vi "LIDAR V2 Mem1 Manager.vi"(11 "Source Name":refnum<k21>="100 MHz Clock") -> ()   [LabVIEW 2013]
uses:
  <vilib>/Platform/TimedLoop/XDataNode/timing_clust.ctl
  <vilib>/Platform/TimedLoop/XDataNode/nitl_modes.ctl
  <vilib>/Platform/TimedLoop/XDataNode/wakeup.ctl
  <vilib>/rvi/DataTransferAndStorage/Container/Common/niFpgaContainerGetUniqueNameForEmu.vi
  <vilib>/rvi/DataTransferAndStorage/Container/Common/niFpgaContainerSetEmuInfo.vi
  <vilib>/rvi/eio/common/nirviEmuReportErrorAndStop.vi
  <vilib>/rvi/Emulation/niFpgaSctlEmulationGetInTimedLoop.vi
  <vilib>/rvi/Emulation/niFpgaEmulationReportErrorSimple.vi
  <vilib>/rvi/Emulation/niFpgaGetClockAttributes.vi
  <vilib>/rvi/Emulation/niFpgaCriticalErrorInLSC.vi
  <vilib>/rvi/DataTransferAndStorage/Container/Common/niFpgaContainerExecOnDevCompGetState.vi
  <vilib>/rvi/FIFO/Fifo_Resource/nirvififoEmulationReadFpgaImpl.vi
  <vilib>/rvi/interface/RandomDataEmulation/nirviRandomDataFPGAFIFO.vi
  <vilib>/rvi/interface/RandomDataEmulation/niFpgaRandomDataHandleErrors.vi
  <vilib>/rvi/Memory/Memory_Emulation/nirvimemoryFastEmulationFpgaImpl.vi
  <instcachedir>/0/nirvimemoryFastEmulationFpgaImpl_5FBAB50466BC4C939F684F8805638BFC.lvgen/nirvimemoryFastEmulationFpgaImpl_5FBAB50466BC4C939F684F8805638BFC_008.vi
  <vilib>/rvi/Memory/Memory_Emulation/nirvimemoryFastEmulation.vi
  <vilib>/rvi/Memory/Memory_Emulation/nirvimemoryEmulation.vi
  <vilib>/rvi/FIFO/Fifo_Resource/nirvififoEmulationWriteFpgaImpl.vi
  <vilib>/Platform/TimedLoop/XDataNode/XDataNode.xnode
  <vilib>/rvi/LocalResourceManager/LocalResourceManager.xnode
  <vilib>/rvi/DataTransferAndStorage/Container/XNode/niFpgaContainer.xnode
  <vilib>/rvi/FIFO/Fifo_Resource/niFpgaFifoEmulationRefIn.vi
  <vilib>/rvi/FIFO/Fifo_Resource/nirvififoEmulationRead.vi
  <vilib>/rvi/FXPMathLib/FxpAdd/XNode/nifxpmath_Add.xnode
  <vilib>/rvi/FIFO/Fifo_Resource/nirvififoEmulationWrite.vi
  <vilib>/Platform/TimedLoop/XDataNode/XDNodeRunTimeDep.lvlib
  <vilib>/rvi/FXPMathLib/sim/FxpSim.dll
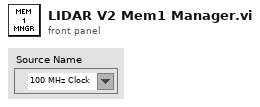
[diagram p1: front panel]
types:
  T1 = typedef "XDNodeRunTimeDep.lvlib/timing_clust.ctl" = cluster{"Expected End [f-1]":u64, "Actual End [f-1]":u64, "Finished Late? [f-1]":bool, "Expected End [i-1]":u64, "Actual End [i-1]":u64, "Finished Late? [i-1]":bool, "Expected Start [i]":u64, "Actual Start [i]":u64, "Expected Start [f]":u64, "Actual Start [f]":u64, "Source Name":string, "Structure Name":string, "Period":i64, "Deadline":i64, "Offset":i64, "Start":i64, "Priority":i32, "Timeout":i32, "Mode":T2, "Wakeup Reason":T3, "Error":errorcluster, "Source Type":string, "Secondary Source Type":string, "Global End Time":u64, "Global Start Time":u64, "Frame Duration":u64, "Iteration Duration":u64, "Assigned CPU":i32, "I/O Scan Engine Mode":u32}
  T2 = typedef "XDNodeRunTimeDep.lvlib/nitl_modes.ctl" = enum32{"No Change", "Process missed periods, maintain original phase", "Discard missed periods, maintain original phase", "Process missed periods, ignore original phase", "Discard missed periods, ignore original phase"}
  T3 = typedef "XDNodeRunTimeDep.lvlib/wakeup.ctl" = enum32{"Normal", "Aborted", "Asynchronous wakeup", "Timing source error", "Timed loop error", "Timeout"}
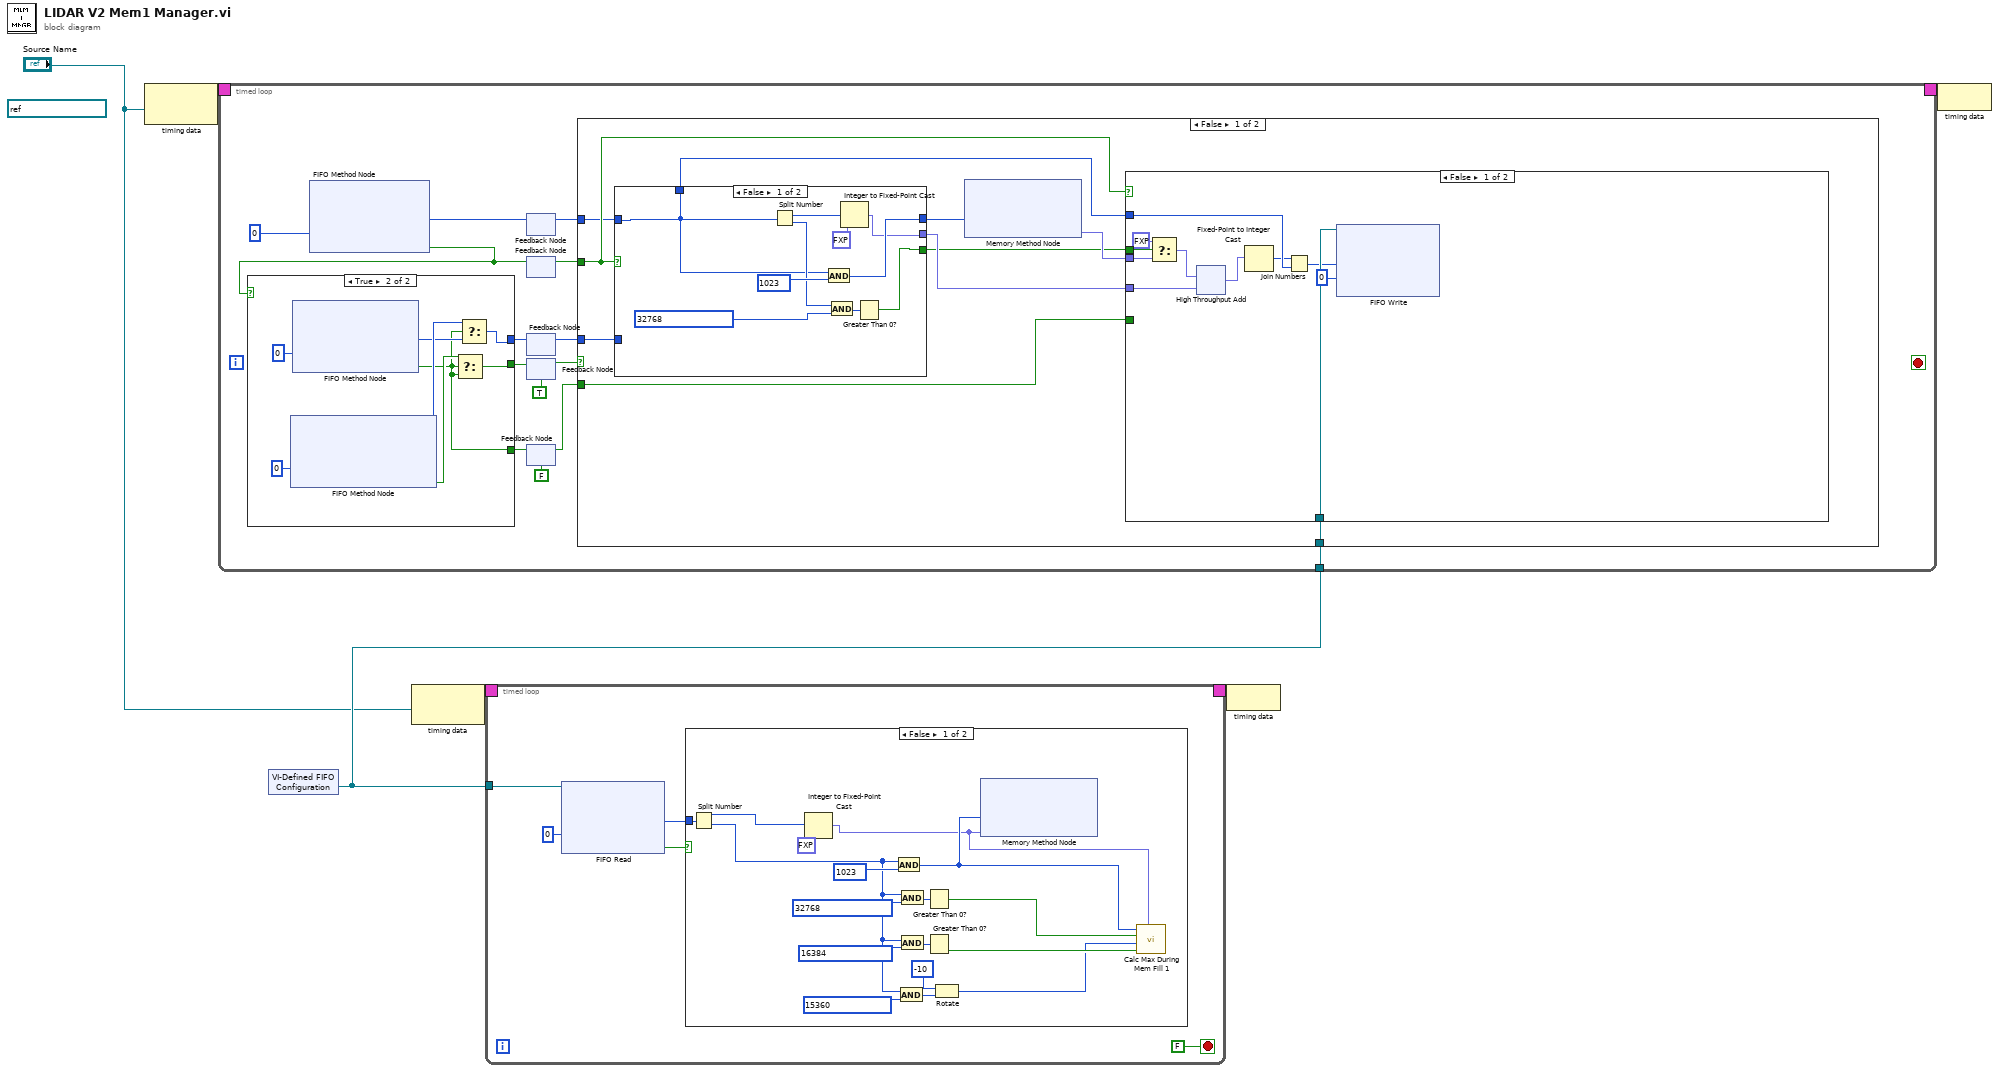
[diagram p0: block diagram]
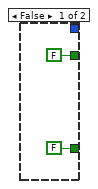
[diagram p3: hidden frame]
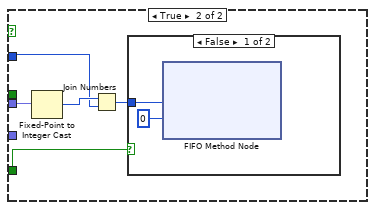
[diagram p4: hidden frame]
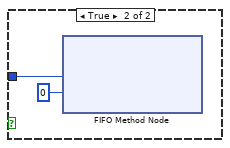
[diagram p5: hidden frame]
diagram:
  (unwired) refnum<k21> "100 MHz Clock" ("Source Name")
  n1 = node-c288("Source Name") -> (w6:T1)
  n2 = xnode "VI-Defined FIFO Configuration"() -> ("FIFO Out"=w4:refnum<k21>)
  n3 = timed-loop {
    timing: w6 -> [_]
    timing-out: [_] -> w5
    tunnel: w4 -> [w15]
    stop <- _ stop-if-true
    n4 = xnode ("FIFO Method Node")("Timeout"=0) -> ("Element"=w20:u32, "Timed Out?"=w17:bool)  [unwired: 1 in, 1 out]
    n5 = case shown="True" w17 {
      tunnel: [FALSE ("Timed Out?") w27] -> w18
      tunnel: [_ w24] -> w16
      tunnel: [FALSE ("Timed Out?") w23] -> w9
      frame False {
      }
      frame True {
        n6 = xnode ("FIFO Method Node")("Timeout"=0) -> ("Element"=w26:u32, "Timed Out?"=w28:bool)  [unwired: 1 in, 1 out]
        n7 = xnode ("FIFO Method Node")("Timeout"=0) -> ("Element"=w25:u32, "Timed Out?"=w23:bool)  [unwired: 1 in, 1 out]
        n8 = Select(t=w28, s=w23, f=w23) -> (s? t:f=w27:bool)
        n9 = Select(t=w26, s=w23, f=w25) -> (s? t:f=w24:u32)
      }
    }
    n10 = feedback-in #1(w20) -> ()
    n11 = feedback #1() -> (w14:u32)  [unwired: 1 in]
    n12 = feedback-in #2(w17) -> ()
    n13 = feedback #2() -> (w13:bool)  [unwired: 1 in]
    n14 = feedback-in #3(w16) -> ()
    n15 = feedback #3() -> (w12:u32)  [unwired: 1 in]
    n16 = feedback-in #4(w18) -> ()
    n17 = feedback #4(TRUE ("Timed Out?")) -> (w11:bool)
    n18 = feedback-in #5(w9) -> ()
    n19 = feedback #5(FALSE ("Timed Out?")) -> (w10:bool)
    n20 = case shown="False" w11 {
      tunnel: w14 -> [w33 _]
      tunnel: w13 -> [w38 _]
      tunnel: w12 -> [w39 _]
      tunnel: w15 -> [w34 _]
      tunnel: w10 -> [w31 _]
      frame False {
        n21 = case shown="False" w38 {
          tunnel: w33 -> [w61 _]
          tunnel: [w64 _] -> w40
          tunnel: [w65 w71] -> w35
          tunnel: w39 -> [_ w71]
          tunnel: [w63 _] -> w36
          tunnel: [w61 w71] -> w32
          frame False {
            n22 = Split Number(x=w61) -> (hi(x)=w70:u16, lo(x)=w62:u16)
            n23 = And(x=w61, y=u32 1023) -> (x .and. y?=w65:u32)
            n24 = And(x=w62, y=u16 32768) -> (x .and. y?=w69:u16)
            n25 = Integer to Fixed-Point Cast(fixed-point type=fxp<+/-,16,16> 0.0, integer=w70) -> (fixed-point=w64:fxp<+/-,16,16>)
            n26 = Greater Than 0?(x=w69) -> (x > 0?=w63:bool)
          }
          frame True {
          }
        }
        n27 = xnode ("Memory Method Node")("Address"=w35) -> ("Data"=w37:fxp<+/-,22,22>)  [unwired: 1 in, 1 out]
        n28 = case shown="False" w38 {
          tunnel: w37 -> [w49 w56]
          tunnel: w40 -> [w51 _]
          tunnel: w32 -> [w44 w53]
          tunnel: w36 -> [w45 _]
          tunnel: w34 -> [w47 _]
          tunnel: w31 -> [_ w52]
          frame False {
            n29 = Select(t=fxp<+/-,22,22> 0.0, s=w45, f=w49) -> (s? t:f=w48:fxp<+/-,22,22>)
            n30 = xnode ("High Throughput Add")("x"=w48, "y"=w51) -> ("x+y"=w46:fxp<+/-,22,22>)
            n31 = Fixed-Point to Integer Cast(1:w46) -> (0:w41:i32)
            n32 = Join Numbers(hi=w41, lo=w44) -> ((hi.lo)=w43:u64)
            n33 = xnode ("FIFO Write")("Element"=w43, "Timeout"=0, "FIFO In"=w47) -> ()  [unwired: 2 out]
          }
          frame True {
            n34 = Fixed-Point to Integer Cast(1:w56) -> (0:w54:i32)
            n35 = Join Numbers(hi=w54, lo=w53) -> ((hi.lo)=w55:u64)
            n36 = case shown="False" w52 {
              tunnel: w55 -> [w57 w59]
              frame False {
                n37 = xnode ("FIFO Method Node")("Element"=w57, "Timeout"=0) -> ()  [unwired: 1 in, 2 out]
              }
              frame True {
                n38 = xnode ("FIFO Method Node")("Element"=w59, "Timeout"=0) -> ()  [unwired: 1 in, 2 out]
              }
            }
          }
        }
      }
      frame True {
      }
    }
  }
  n39 = node-c288("Source Name") -> (w3:T1)
  n40 = timed-loop {
    tunnel: w4 -> [w76]
    timing: w3 -> [_]
    timing-out: [_] -> w2
    stop <- FALSE stop-if-true
    n41 = xnode ("FIFO Read")("Timeout"=0, "FIFO In"=w76) -> ("Element"=w78:u64, "Timed Out?"=w74:bool)  [unwired: 1 out]
    n42 = case shown="False" w74 {
      tunnel: w78 -> [w95 _]
      frame False {
        n43 = Split Number(x=w95) -> (hi(x)=w86:u32, lo(x)=w85:u32)
        n44 = Integer to Fixed-Point Cast(fixed-point type=fxp<+/-,22,22> 0.0, integer=w86) -> (fixed-point=w83:fxp<+/-,22,22>)
        n45 = And(x=w85, y=u32 1023) -> (x .and. y?=w84:u32)
        n46 = And(x=w85, y=u32 15360) -> (x .and. y?=w81:u32)
        n47 = And(x=w85, y=u32 32768) -> (x .and. y?=w89:u32)
        n48 = And(x=w85, y=u32 16384) -> (x .and. y?=w88:u32)
        n49 = Greater Than 0?(x=w89) -> (x > 0?=w93:bool)
        n50 = Greater Than 0?(x=w88) -> (x > 0?=w82:bool)
        n51 = Rotate(1:w81, 2:i8 -10 ("x")) -> (0:w80:u32)
        n52 = xnode ("Memory Method Node")("Address"=w84, "Data"=w83) -> ()  [unwired: 1 in, 1 out]
        n53 = call "Calc Max During Mem Fill 1.vi"("Value"=w83, "LastIterration"=w82, "ActiveLedIndex"=w80, "FirstIterration"=w93, "Address"=w84) -> ()  [unwired: 7 in]
      }
      frame True {
      }
    }
  }
  n54 = node-c288(w2) -> ()
  n55 = node-c288(w5) -> ()
